vi "Test - Serial Device - Read Pin 1.vi"(8 "error in (no error)":errorcluster, 11 "Module ID":i32) -> (0 "error out":errorcluster, 3 "Pass":bool)   [LabVIEW 2020]
doc: "_____\nCreated using Delacor QMH Event Scripter 5.0.0.112."
uses:
  Libraries/Serial Device/Serial Device.lvlib
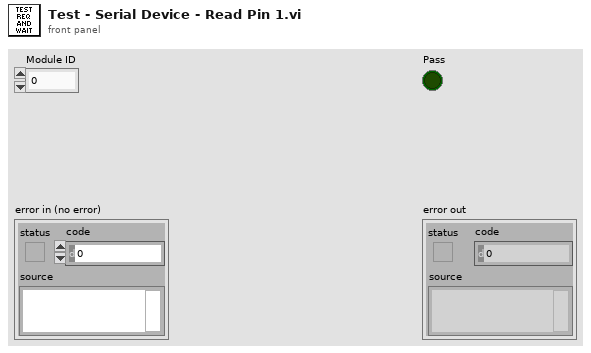
[diagram p1: front panel]
types:
  T1 = typedef "Serial Device.lvlib/Read Pin (Reply Payload)--cluster.ctl" = cluster{"Read Pin_error":errorcluster, "Response":string}
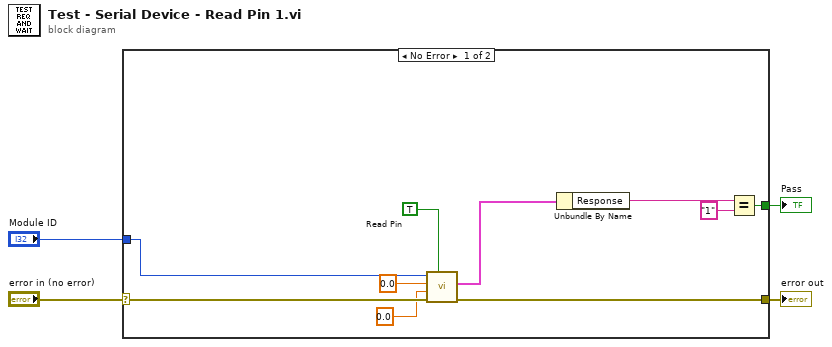
[diagram p0: block diagram]
diagram:
  n1 = case shown="No Error" "error in (no error)" {
    selector: "error in (no error)" -> [w14 w15]
    tunnel: [w13 w15] -> w3
    tunnel: "Module ID" -> [w12 _]
    tunnel: [w11 _] -> w1
    frame No Error {
      n2 = call "Read Pin.vi"("Pin Value"=TRUE, "error in (no error)"=w14, "Pin 2"=0.0, "Port 4"=0.0, "Module ID"=w12) -> ("error out"=w13:errorcluster, "Reply Payload"=w10:T1)  [unwired: 4 in, 1 out]
      n3 = Unbundle By Name(w10) -> ("Response"=w9:string)
      n4 = Equal?(x=w9, y="1") -> (x = y?=w11:bool)
    }
    frame Error {
    }
  }
  "error out" <- w3
  "Pass" <- w1
